vi "Create Channel.vi"(6 "index":i32, 8 "error in":errorcluster, 10 "channel settings":T1, 11 "digital output mode in":refnum<class "Digital Output Mode.lvclass">) -> (0 "error out":errorcluster, 2 "digital output channel":refnum<class "DO Channel.lvclass">, 3 "digital output mode out":refnum<class "Digital Output Mode.lvclass">)   [LabVIEW 2020, in "Scan Engine Scripting.lvlib" / "Digital Output Mode.lvclass"]
uses:
  Digital Output Mode.lvclass
  Controls/digital channel settings.ctl
  Channel Classes/DO Channel/DO Channel.lvclass
  Digital Output Mode.lvclass/Digital Output Mode.ctl
  Scan Engine Scripting.lvlib
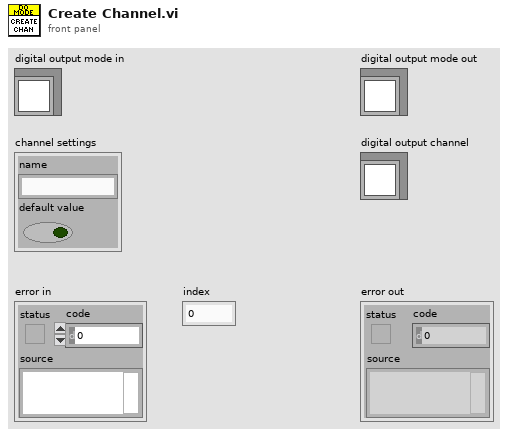
[diagram p1: front panel]
types:
  T1 = typedef "Scan Engine Scripting.lvlib/digital channel settings.ctl" = cluster{"name":string, "default value":bool}
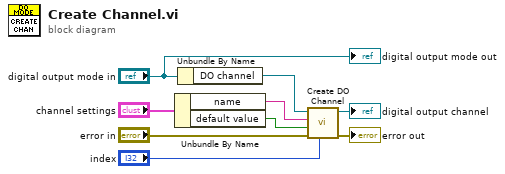
[diagram p0: block diagram]
diagram:
  n1 = Unbundle By Name("channel settings") -> ("name"=w1:string, "default value"=w2:bool)
  n2 = Unbundle By Name("digital output mode in") -> ("DO channel"=w3:refnum<class "DO Channel.lvclass">)
  n3 = call-dynamic "Create DO Channel.vi"("index"="index", "error in"="error in", "default value"=w2, "name"=w1, "DO channel in"=w3) -> ("error out"=→"error out":errorcluster, "DO channel out"=→"digital output channel":refnum<class "DO Channel.lvclass">)  [unwired: 5 in]
  "digital output mode out" <- "digital output mode in"
